vi "Send Get Bounds and Position.vi"(7 "Message Priority (Normal)":T4=enum."Normal", 8 "error in (no error)":errorcluster, 10 "timeout in ms (100)":i32=100, 11 "Message Enqueuer":refnum<class "Message Enqueuer.lvclass">) -> (0 "error out":errorcluster, 1 "timed out?":bool, 2 "Panel Bounds":T3, 3 "Message Enqueuer out":refnum<class "Message Enqueuer.lvclass">, 4 "Panel Position":T1, 5 "Actor Name":string, 6 "Windows Bounds":T2)   [LabVIEW 2014, in "ViewableActor.lvlib" / "Get Bounds and Position Msg.lvclass"]
doc: "This VI sends the message to an actor."
uses:
  Get Bounds and Position Msg.lvclass
  <vilib>/ActorFramework/Message Enqueuer/Message Enqueuer.lvclass
  <vilib>/ActorFramework/Message Enqueuer/Message Priority.ctl
  <vilib>/Utility/miscctls.llb/LVBoundsTypeDef.ctl
  <vilib>/Utility/miscctls.llb/LVRectTypeDef.ctl
  <vilib>/Utility/miscctls.llb/LVPositionTypeDef.ctl
  <vilib>/ActorFramework/Reply Msg/Reply Msg.lvclass/Reply Msg.ctl
  <vilib>/ActorFramework/Message Enqueuer/Message Enqueuer.lvclass/Message Enqueuer.ctl
  <vilib>/ActorFramework/Message Enqueuer/Enqueue.vi
  <vilib>/ActorFramework/Message Priority Queue/Priority Enqueue.vi
  <vilib>/ActorFramework/Reply Msg/Reply Msg.lvclass
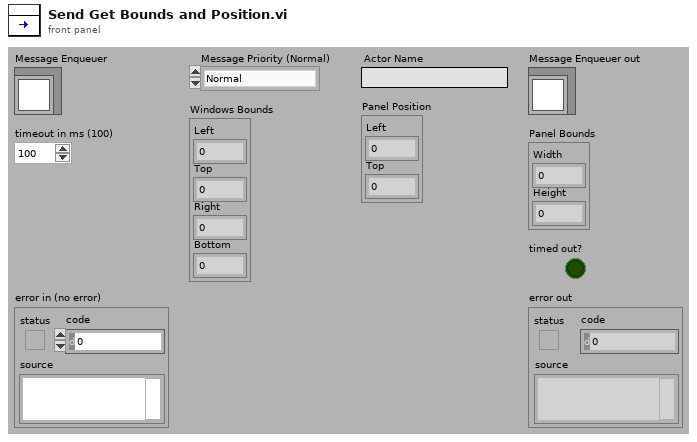
[diagram p1: front panel]
types:
  T1 = typedef "LVPositionTypeDef.ctl" = cluster{"Left":i32, "Top":i32}
  T2 = typedef "LVRectTypeDef.ctl" = cluster{"Left":i16, "Top":i16, "Right":i16, "Bottom":i16}
  T3 = typedef "LVBoundsTypeDef.ctl" = cluster{"Width":u32, "Height":u32}
  T4 = typedef "Actor Framework.lvlib/Message Enqueuer.lvclass/Message Priority.ctl" = enum16{"Low", "Normal", "High"}
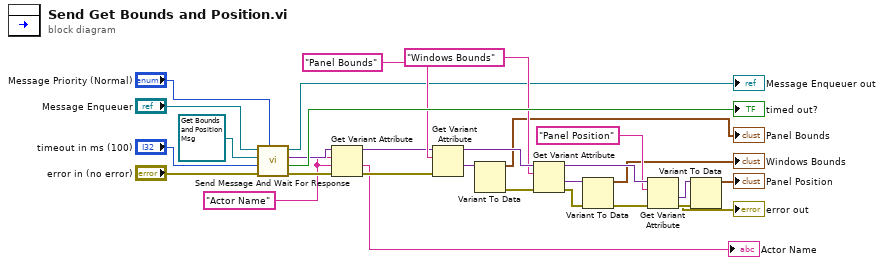
[diagram p0: block diagram]
diagram:
  w2 = "Actor Name" ("name")
  n1 = call <vilib>:"Send Message And Wait For Response.vi"("Message Priority (Normal)"="Message Priority (Normal)", "error in (no error)"="error in (no error)", "timeout in ms (-1)"="timeout in ms (100)", "Original Message"=refnum<class "Get Bounds and Position Msg.lvclass"> refnum ("Object"), "Message Enqueuer in"="Message Enqueuer") -> ("error out"=w4:errorcluster, "timed out?"=→"timed out?":bool, "Reply"=w6:variant, "Message Enqueuer out"=→"Message Enqueuer out":refnum<class "Message Enqueuer.lvclass">)  [unwired: 3 in]
  n2 = Get Variant Attribute(Variant=w6, name=w2, default value (empty Variant)=w2, error in=w4) -> (duplicate Variant=w5:variant, value=→"Actor Name":string, error out=w3:errorcluster)  [unwired: 1 out]
  n3 = Get Variant Attribute(Variant=w5, name="Panel Bounds", error in=w3) -> (duplicate Variant=w23:variant, value=w18:variant)  [unwired: 1 in, 2 out]
  n4 = Variant To Data(Variant=w18) -> (data=→"Panel Bounds":T3, error out=w15:errorcluster)  [unwired: 2 in]
  n5 = Get Variant Attribute(Variant=w23, name="Windows Bounds", error in=w15) -> (duplicate Variant=w22:variant, value=w17:variant, error out=w14:errorcluster)  [unwired: 1 in, 1 out]
  n6 = Variant To Data(error in=w14, Variant=w17) -> (data=→"Windows Bounds":T2, error out=w13:errorcluster)  [unwired: 1 in]
  n7 = Get Variant Attribute(Variant=w22, name="Panel Position", error in=w13) -> (value=w8:variant, error out=w12:errorcluster)  [unwired: 1 in, 2 out]
  n8 = Variant To Data(error in=w12, Variant=w8) -> (data=→"Panel Position":T1, error out=→"error out":errorcluster)  [unwired: 1 in]
